vi "Update Method Getter.vi"(5 "Library":refnum<vi>, 7 "RPC Method Name":string, 8 "error in (no error)":errorcluster, 10 "Request Metadata Name":string, 11 "Server class in":refnum<vi>) -> (0 "error out":errorcluster, 3 "Server class out":refnum<vi>)   [LabVIEW 2019, in "gRPC Template Creation Utility.lvlib"]
uses:
  gRPC Template Creation Utility.lvlib
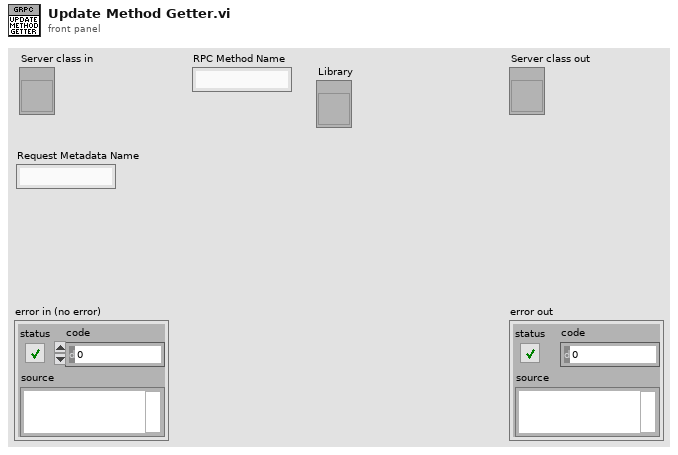
[diagram p1: front panel]
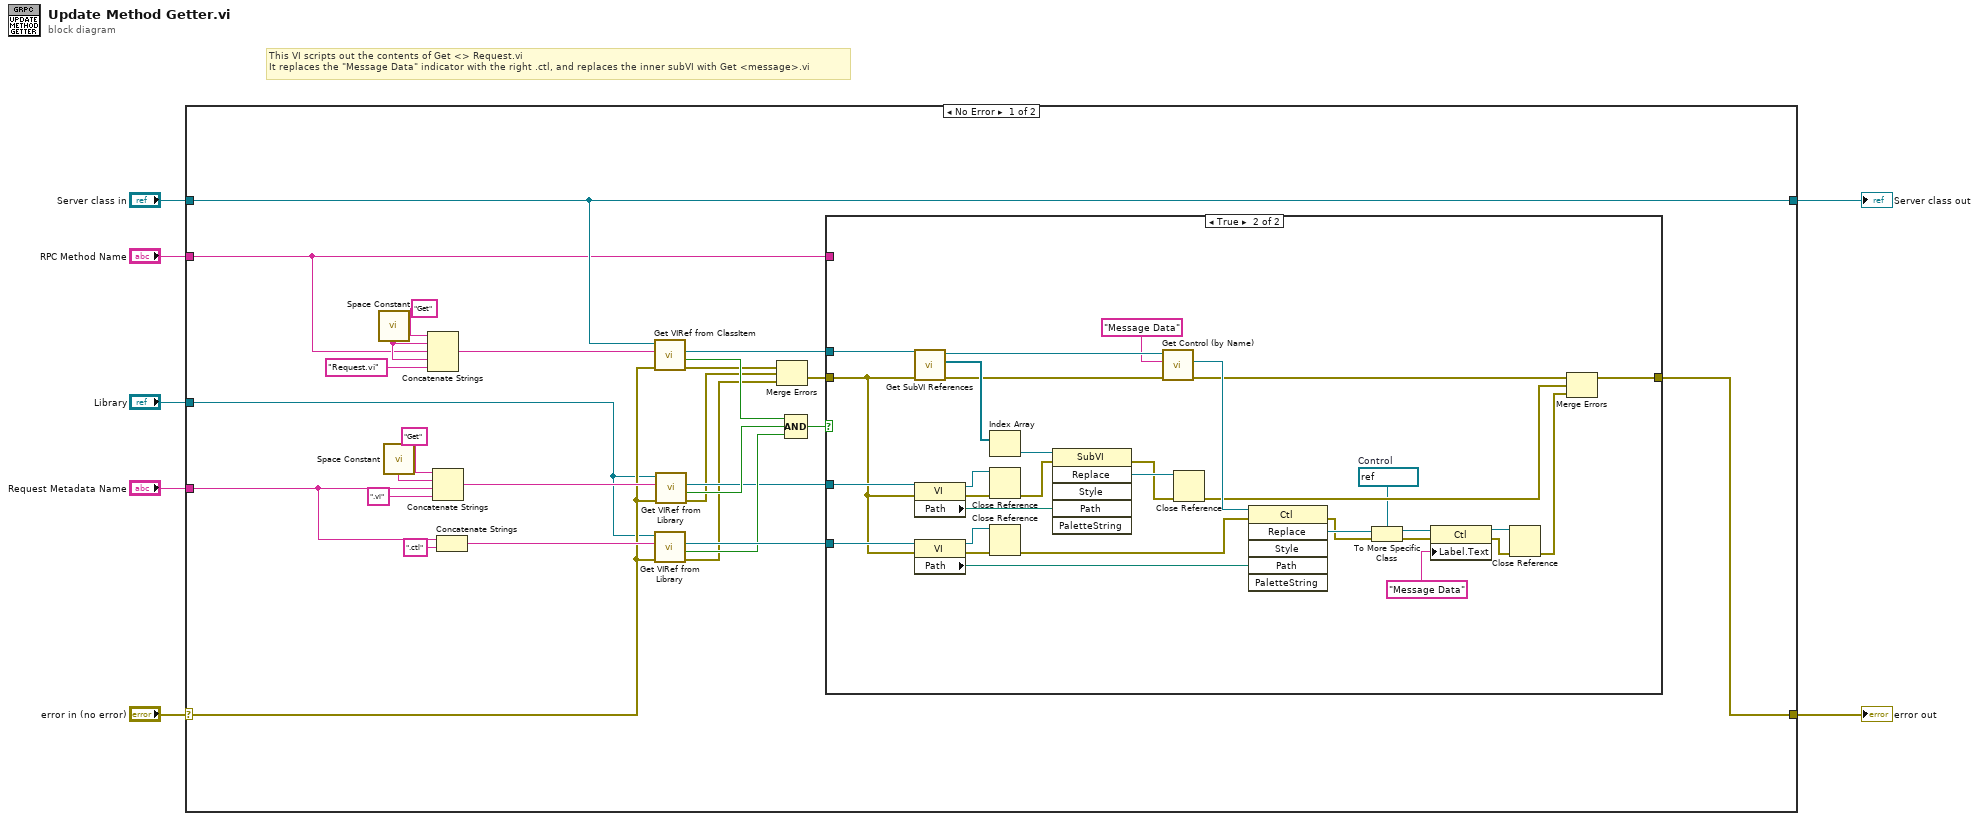
[diagram p0: block diagram]
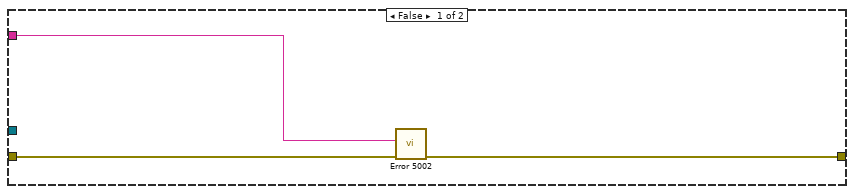
[diagram p2: hidden frame]
diagram:
  # "This VI scripts out the contents of Get <> Request.vi\nIt replaces the \"Message Data\" indicator with the right .ctl, and replaces the inner subVI with Get <message>.vi"
  n1 = case shown="No Error" "error in (no error)" {
    selector: "error in (no error)" -> [w16 w71]
    tunnel: "Server class in" -> [w10 w70]
    tunnel: "Request Metadata Name" -> [w27 _]
    tunnel: "RPC Method Name" -> [w9 _]
    tunnel: [w11 w71] -> w3
    tunnel: [w10 w70] -> w2
    tunnel: "Library" -> [w8 _]
    frame No Error {
      n2 = call <vilib>:"Space Constant.vi"() -> ("String"=w18:string)
      n3 = call <vilib>:"Space Constant.vi"() -> ("String"=w20:string)
      n4 = Concatenate Strings("Get" ("string"), w18, w9, w18, "Request.vi" ("string")) -> (w24:string)
      n5 = Concatenate Strings("Get" ("string"), w20, w27, ".vi" ("string")) -> (w23:string)
      n6 = Concatenate Strings(w27, ".ctl" ("string")) -> (w29:string)
      n7 = call "Get VIRef from ClassItem.vi"("error in (no error)"=w16, "Item Name"=w24, "LVClassLibrary in"=w10) -> ("error out"=w15:errorcluster, "Found ?"=w30:bool, "VIref out"=w25:refnum<vi>)  [unwired: 5 in, 1 out]
      n8 = call "Get VIRef from Library.vi"("error in (no error)"=w16, "Item Name"=w29, "Library"=w8) -> ("error out"=w12:errorcluster, "Found ?"=w32:bool, "VIref out"=w34:refnum<vi>)  [unwired: 5 in, 1 out]
      n9 = call "Get VIRef from Library.vi"("error in (no error)"=w16, "Item Name"=w23, "Library"=w8) -> ("error out"=w13:errorcluster, "Found ?"=w31:bool, "VIref out"=w26:refnum<vi>)  [unwired: 5 in, 1 out]
      n10 = Merge Errors(w15, w13, w12) -> (w14:errorcluster)
      n11 = Compound Arithmetic op=AND(w30, w31, w32) -> (w33:bool)
      n12 = case shown="True" w33 {
        tunnel: w25 -> [_ w67]
        tunnel: w26 -> [_ w66]
        tunnel: w34 -> [_ w62]
        tunnel: w14 -> [w37 w56]
        tunnel: [w36 w38] -> w11
        tunnel: w9 -> [w35 _]
        frame False {
          n13 = call "Error 5002.vi"("error in (no error)"=w37, "Method Name"=w35) -> ("error out"=w36:errorcluster)  [unwired: 9 in]
        }
        frame True {
          w45 = refnum<vi> refnum  # Control
          n14 = call "Get SubVI References.vi"("error in (no error)"=w56, "Owner vi in"=w67) -> ("error out"=w57:errorcluster, "SubVI refs"=w69:refnum<vi>[], "Owner vi out"=w60:refnum<vi>)  [unwired: 7 in]
          n15 = property class="VI"(reference=w66, error in=w56) -> (reference out=w52:refnum<vi>, error out=w53:errorcluster, "Path"=w65:path)
          n16 = property class="VI"(reference=w62, error in=w56) -> (reference out=w50:refnum<vi>, error out=w51:errorcluster, "Path"=w61:path)
          n17 = Index Array(array=w69) -> (element=w68:refnum<vi>)  [unwired: 1 in]
          n18 = Close Reference(reference=w52, error in (no error)=w53) -> (error out=w48:errorcluster)
          n19 = Close Reference(reference=w50, error in (no error)=w51) -> (error out=w49:errorcluster)
          n20 = invoke class="SubVI" method="Replace"(reference=w68, error in=w48, "Path"=w65) -> (error out=w63:errorcluster, "Replace"=w64:refnum<vi>)  [unwired: 3 in, 4 out]
          n21 = call "Get Control (by Name).vi"("error in (no error)"=w57, "Control Label"="Message Data" ("Constant Label"), "Owner VI in"=w60) -> ("error out"=w55:errorcluster, "Control Refnum"=w58:refnum<vi>)  [unwired: 5 in, 2 out]
          n22 = Close Reference(reference=w64, error in (no error)=w63) -> (error out=w54:errorcluster)
          n23 = invoke class="Ctl" method="Replace"(reference=w58, error in=w49, "Path"=w61) -> (error out=w46:errorcluster, "Replace"=w47:refnum<vi>)  [unwired: 3 in, 4 out]
          n24 = To More Specific Class(target class=w45, reference=w47, error in=w46) -> (specific class reference=w43:refnum<vi>, error out=w44:errorcluster)
          n25 = property class="Ctl"(reference=w43, error in=w44, "Label.Text"="Message Data") -> (reference out=w40:refnum<vi>, error out=w41:errorcluster)
          n26 = Close Reference(reference=w40, error in (no error)=w41) -> (error out=w39:errorcluster)
          n27 = Merge Errors(w55, w54, w39) -> (w38:errorcluster)
        }
      }
    }
    frame Error {
    }
  }
  "Server class out" <- w2
  "error out" <- w3
